vi "CV.vi"(2 "Run uninterrupted?":bool, 3 "Device Category IN:":string(combo)="Short Strip" caption="Device Category:", 4 "Batch No.:":string, 5 "Wafer Serial No.:":string, 6 "Sensor Serial No.:":string) -> (0 "Done!":bool)   [LabVIEW 2018]
doc: "Performs CV measurements according to ATLAS ITk Quality Control Specifications."
uses:
  general_VIs/globals/QC_MeasurementSetup.vi
  general_VIs/globals/QC_RunInformation.vi
  InstrControl/InstrumentSetup.vi
  InstrControl/Switching/Switching.lvclass
  InstrControl/SupplyControl/SupplyControl.lvclass
  InstrControl/LCRControl/LCRControl.lvclass
  InstrControl/ArduinoControl/ArduinoControl.lvclass
  <vilib>/Analysis/NI_AALBase.lvlib
  InstrControl/InstrControl.lvclass
panel:
  out "Frequency [Hz]":i32=1000 format="%#.3p"
  out "Resistance":dbl[](array[numeric]) caption="Res [kOhm]"
  out "Initial volts [V]":dbl format="%.1f"
  out "Final volts [V]":dbl=-700.0 format="%.1f"
  out "step [V]":dbl=10.0 format="%.1f"
  out "step interval [s]":u32=5
  out "Volts":dbl[](array[numeric]) caption="Volts [V]"
  out "Capacitance":dbl[](array[numeric]) caption="Cap [pF]"
  out "Temp.":dbl[](array[numeric]) caption="Temp. [°C]" format="%#.2f"
  out "RH":dbl[](array[numeric]) caption="RH [%]" format="%#.2f"
  out "Cgraph":cluster{"Initial volts":dbl, dbl, dbl[]}(graph)
  in  "Scales":T1(ring)
  in  "Cscale":enum16{"1/C^2 [1/nF^2]", "nF", "pF"}(ring)
  out "positive ramp?":bool
  out "Tab Control":enum32{"CV Setup", "CV Scan"}(tab)
  in  "Switching":string(combo)="LXIPXI Switching"
  in  "Frequency [Hz] Setup":i32=1000 caption="Frequency [Hz]" format="%#.3p"
  in  "LCR Meter":string(combo)="WayneKerr 6440B"
  in  "User:":string(combo)="Graham"
  in  "CV Supply":string(combo)="Keithley 2410"
  in  "Configurations":bool
  in  "Set\ncurrent\nlimit?":bool
  in  "Current \nLimit \n[µA]":dbl=1000.0 min=0.0001 format="%.3f"
  in  "Manufacturer:":string(combo)="Hamamatsu"
  in  "Quit":bool
  in  "Continue":bool
  in  "Temperature":enum16{"Read Arduino", "Enter manually"}(ring)=enum."Enter manually"
  in  "abort":bool
  out "Device Category:":string
  out "Batch:":string
  out "Current Volts:":dbl format="%.2f"
  in  "quit (no save)":bool
  in  "Quit & Save":bool
  out "Bias On/Off:":bool
  out "STATUS 1":string
  out "Initiated:":string
  out "Sensor No.:":string
  out "No of steps":u32
  out "Current reading No.":u32
  out "Last reading at:":string
  # "University of\nCambridge"
  # "Strip Sensor QC: CV"
  # "CV Scan parameters:"
  # "Last 5 readings:"
  # "n-4"
  # "n-3"
  # "n-2"
  # "n-1"
  # "n"
  # "Vertical Scale:"
  # "DUT & Test Description"
  # "Hardware"
  # "DUT & Test Description:"
  # "Current status:"
  # "Rdg No:"
  # "out of"
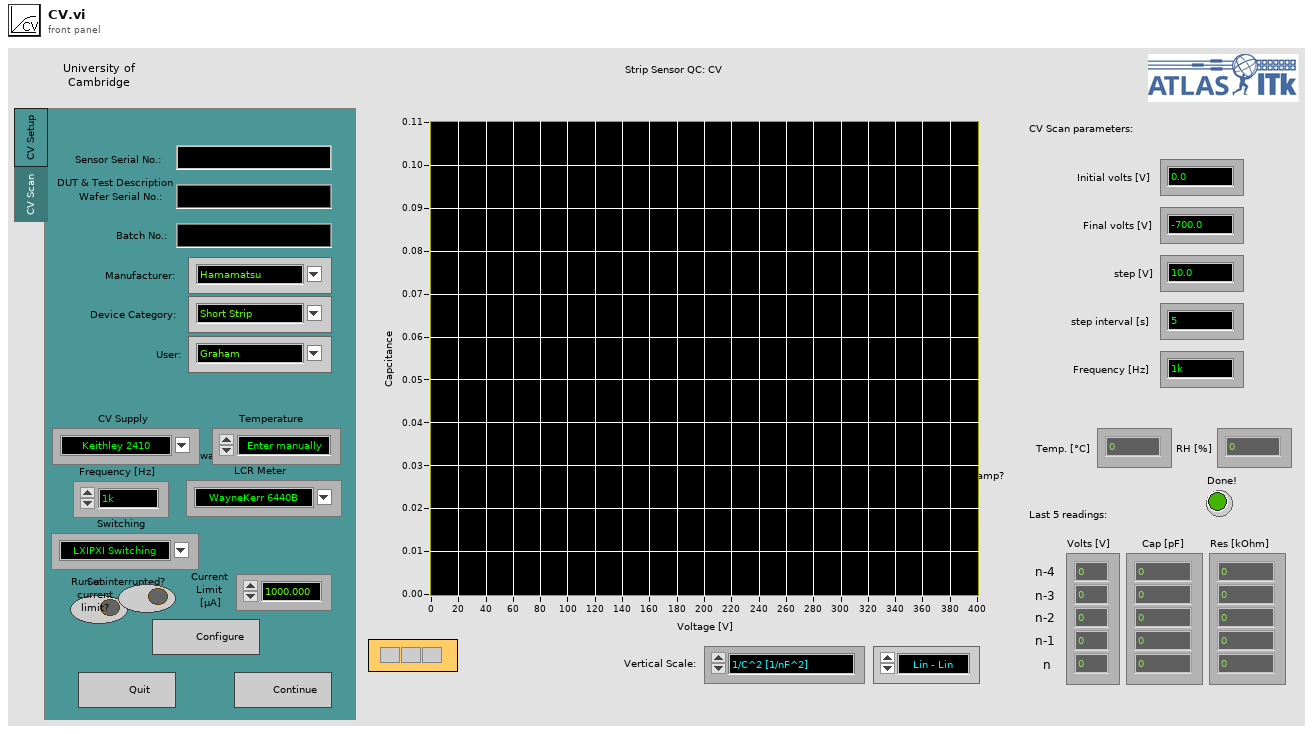
[diagram p1: front panel]
types:
  T1 = enum16{"Lin - Lin", "Log - Lin", "Lin - Log", "Log - log"}
  T2 = enum32{"IV", "CV", "Stability", "Striptest", "Cis", "Ris", "PTP"}
  T3 = enum16{"Reset", "Read Array", "Read Element", "Write Element", "Write Array", "Add Element", "Add Array"}
  T4 = enum16{"Reset", "Ground", "Striptest SMU", "Striptest LCR", "IV", "CV", "Interstrip Cap", "Interstrip Res"}
  T5 = cluster{"Sensor Serial No.:":string, "Wafer Serial No.:":string, "Batch:":string, "Manufacturer:":string, "Device Category:":string, "Database Serial No.:":string, "Initiated:":string, "Test":string, "Instruments used:":string, "Probeplan used:":string, "End of Run comment:":string, "User:":string}
  T6 = cluster{"Institute":string, "Manufacturers":string[], "Devices":string[], "Serialnumbers Lookup DB":string, "Data directory":string, "Backup & screenshot directory":string, "List of known users":string[]}
  T7 = cluster{"Supply":refnum<class "SupplyControl.lvclass">, "LCR":refnum<class "LCRControl.lvclass">, "Initial Voltage [V]":dbl, "Final Voltage [V]":dbl, "Step Size [V]":dbl, "Step Interval [s]":i32, "Number Of Steps":u32, "AC frequency [Hz]":i32, "RC Configuration":u16, "AC amplitude [V]":dbl, "Ramp down steps [V]":dbl, "Ramp down Interval [s]":i32, "Set Current Limit?":bool, "Current Limit [µA]":dbl, "Temperature Readout":enum16{"Read Arduino", "Enter manually"}, "Arduino":refnum<class "ArduinoControl.lvclass">, "Supply Name":string, "LCR Name":string, "V_depletion Limit [V]":dbl, "Switching":refnum<class "Switching.lvclass">}
  T8 = cluster{"VISA address":refnum<visa-resource-name>, "T sensor":enum16{"SHT", "DS"}, "Arduino":refnum<class "ArduinoControl.lvclass">}
  T9 = cluster{"Matrix address":string, "Mux1 address":string, "Mux2 address":string, "Matrix used?":bool, "Switching":refnum<class "Switching.lvclass">, "Matrix X Channels":cluster{"Bias Supply / SMU LO":i32, "Bias Supply / SMU HI":i32, "CV Box LO":i32, "CV Box HI":i32, "CV Box LO IN":i32, "CV Box HI IN":i32, "Volt meter LO":i32, "Volt meter HI":i32, "Mux1 C1":i32, "Mux1 C2":i32, "Mux2 C1":i32, "Mux2 C2":i32}}
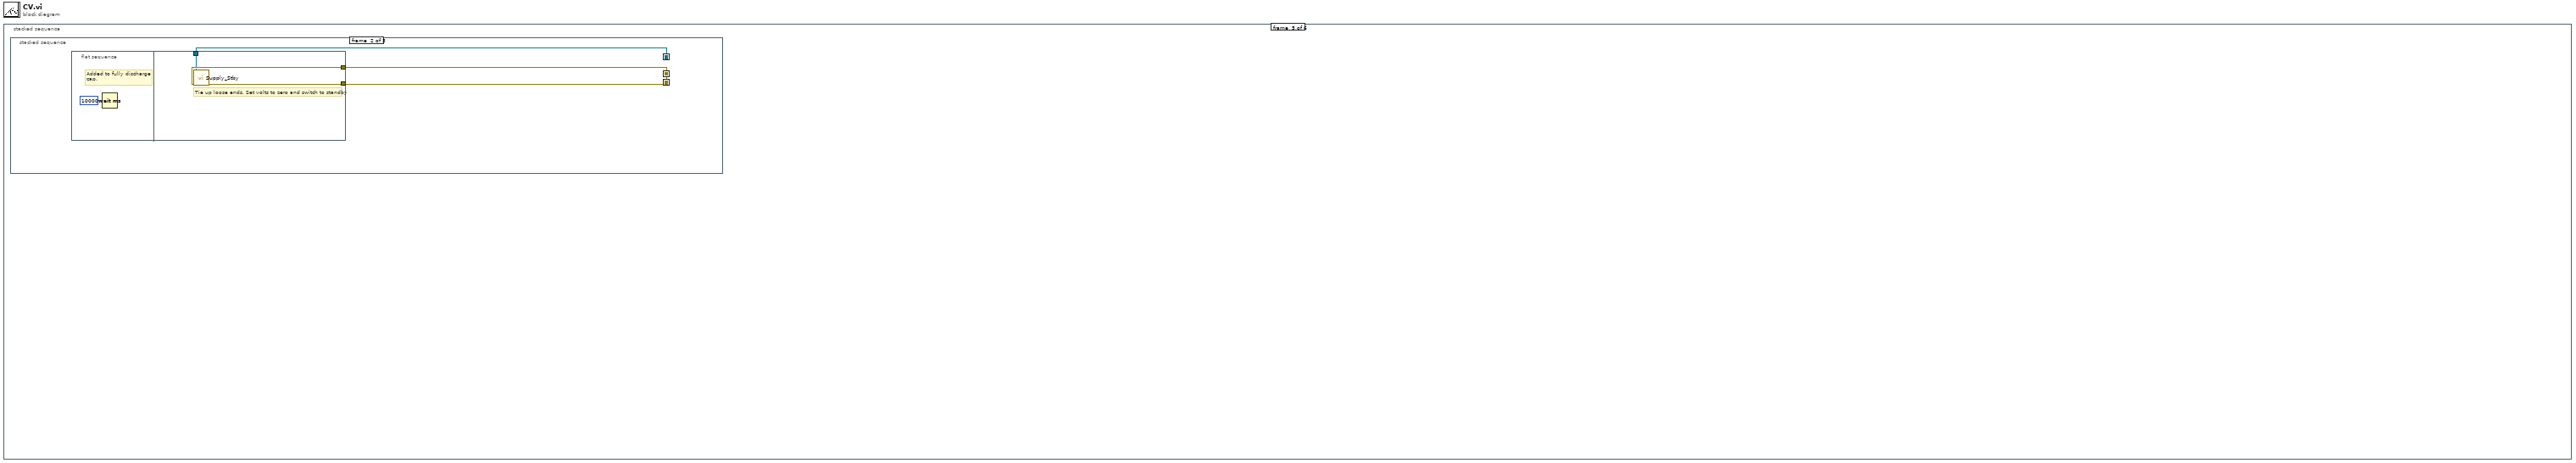
[diagram p0: block diagram]
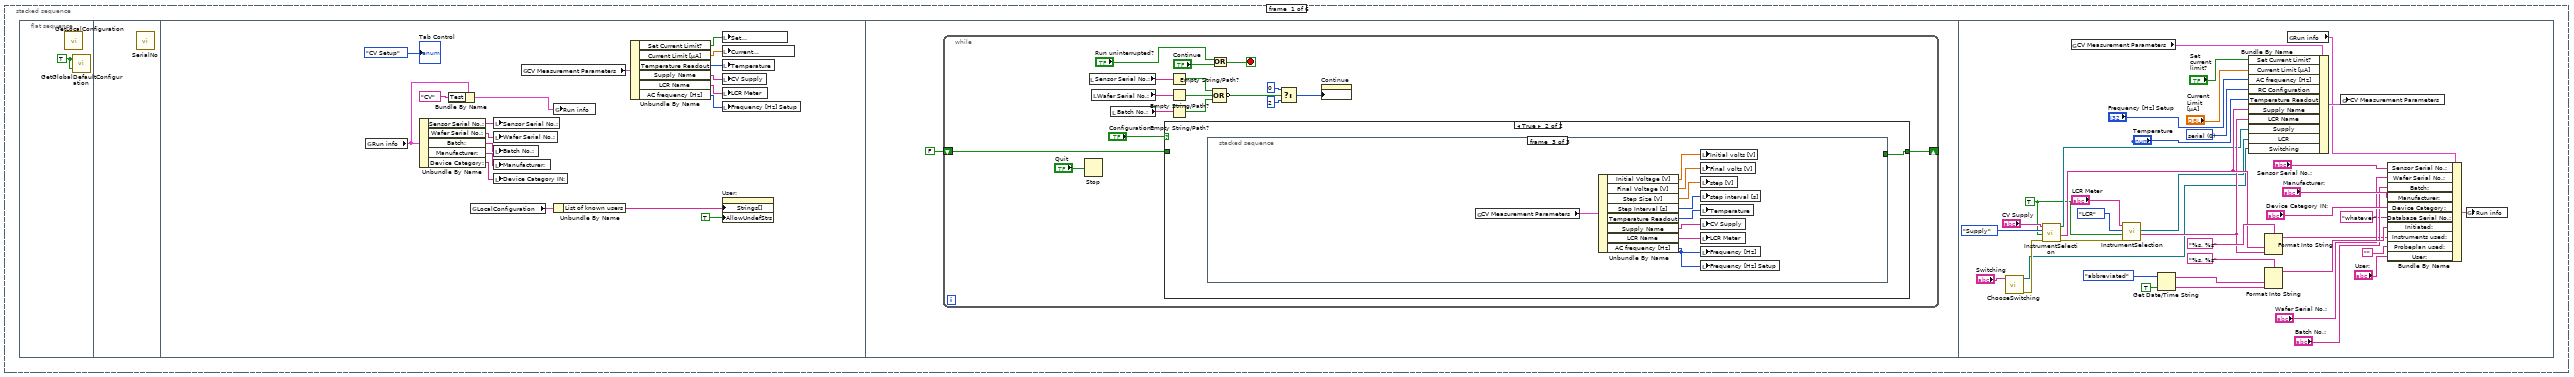
[diagram p2: hidden frame]
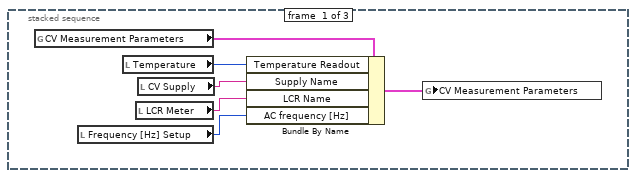
[diagram p4: hidden frame]
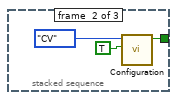
[diagram p5: hidden frame]
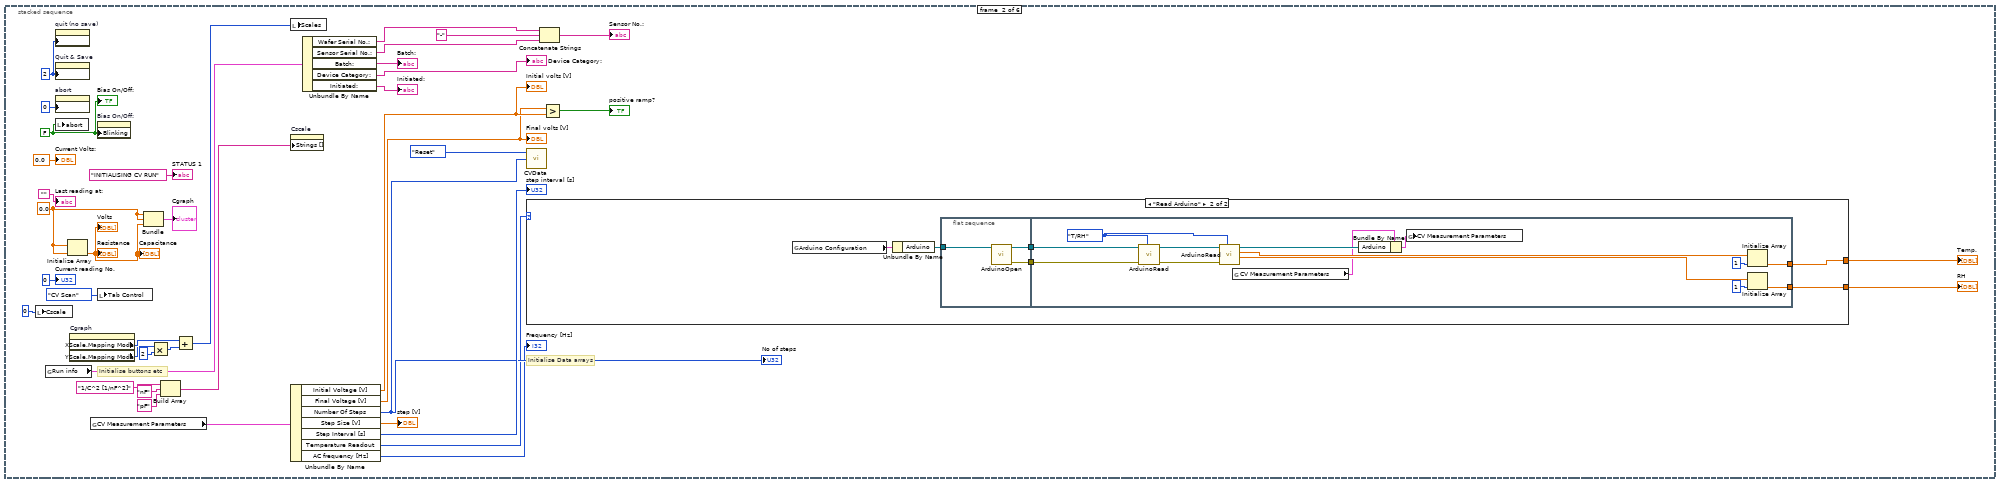
[diagram p6: hidden frame]
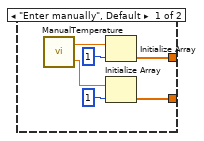
[diagram p7: hidden frame]
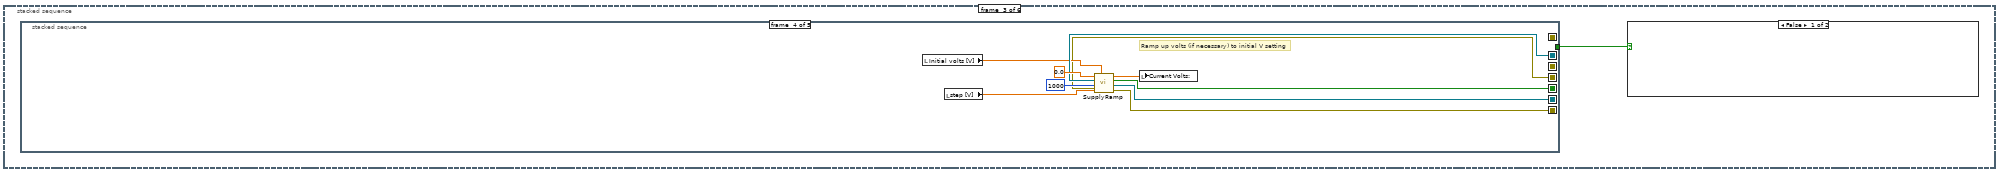
[diagram p8: hidden frame]
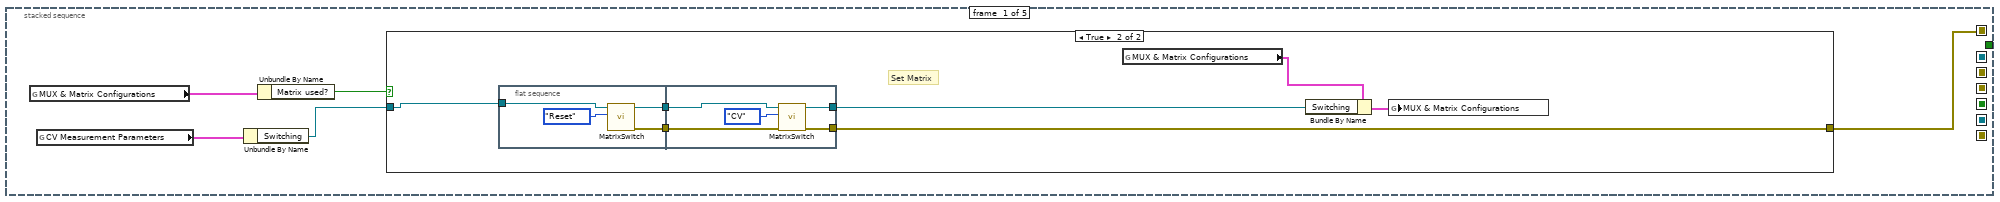
[diagram p9: hidden frame]
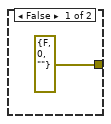
[diagram p10: hidden frame]
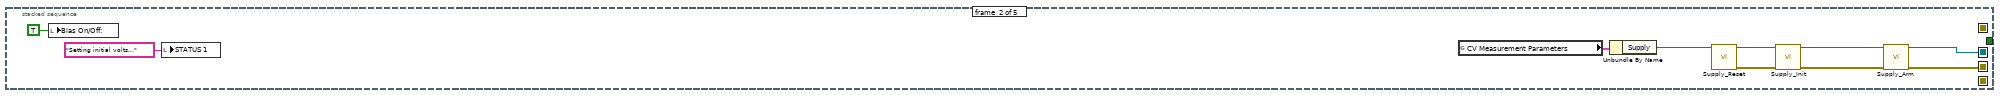
[diagram p11: hidden frame]
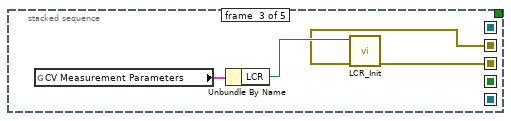
[diagram p12: hidden frame]
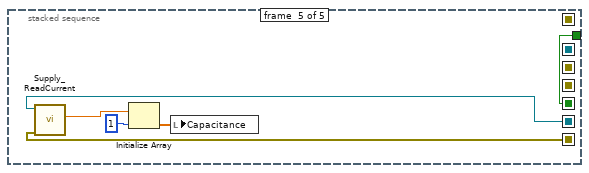
[diagram p13: hidden frame]
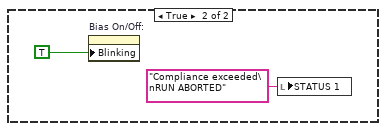
[diagram p14: hidden frame]
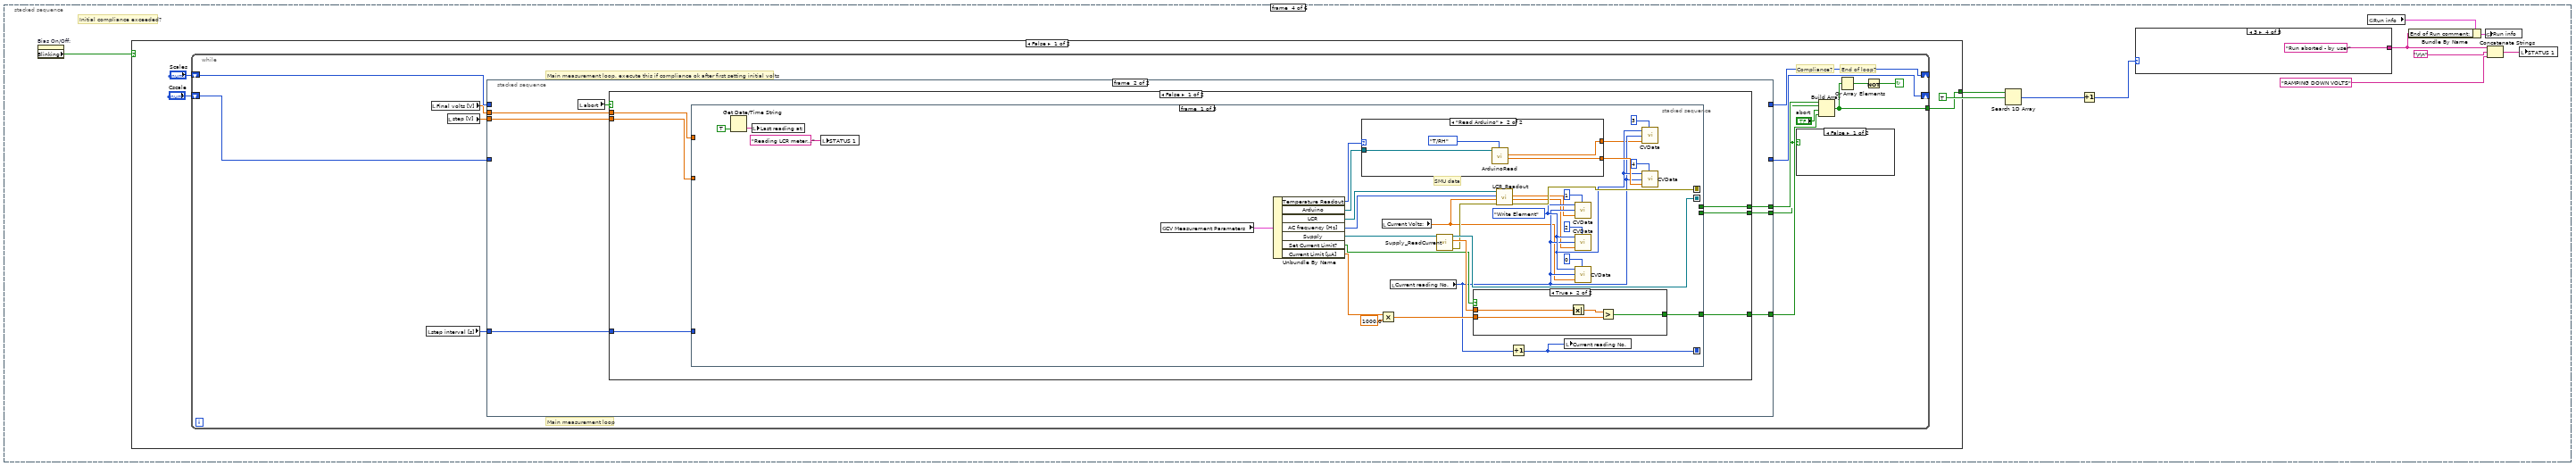
[diagram p15: hidden frame]
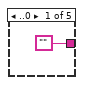
[diagram p16: hidden frame]
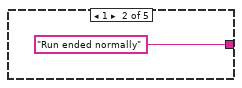
[diagram p17: hidden frame]
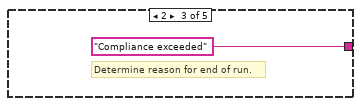
[diagram p18: hidden frame]
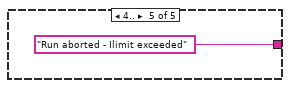
[diagram p19: hidden frame]
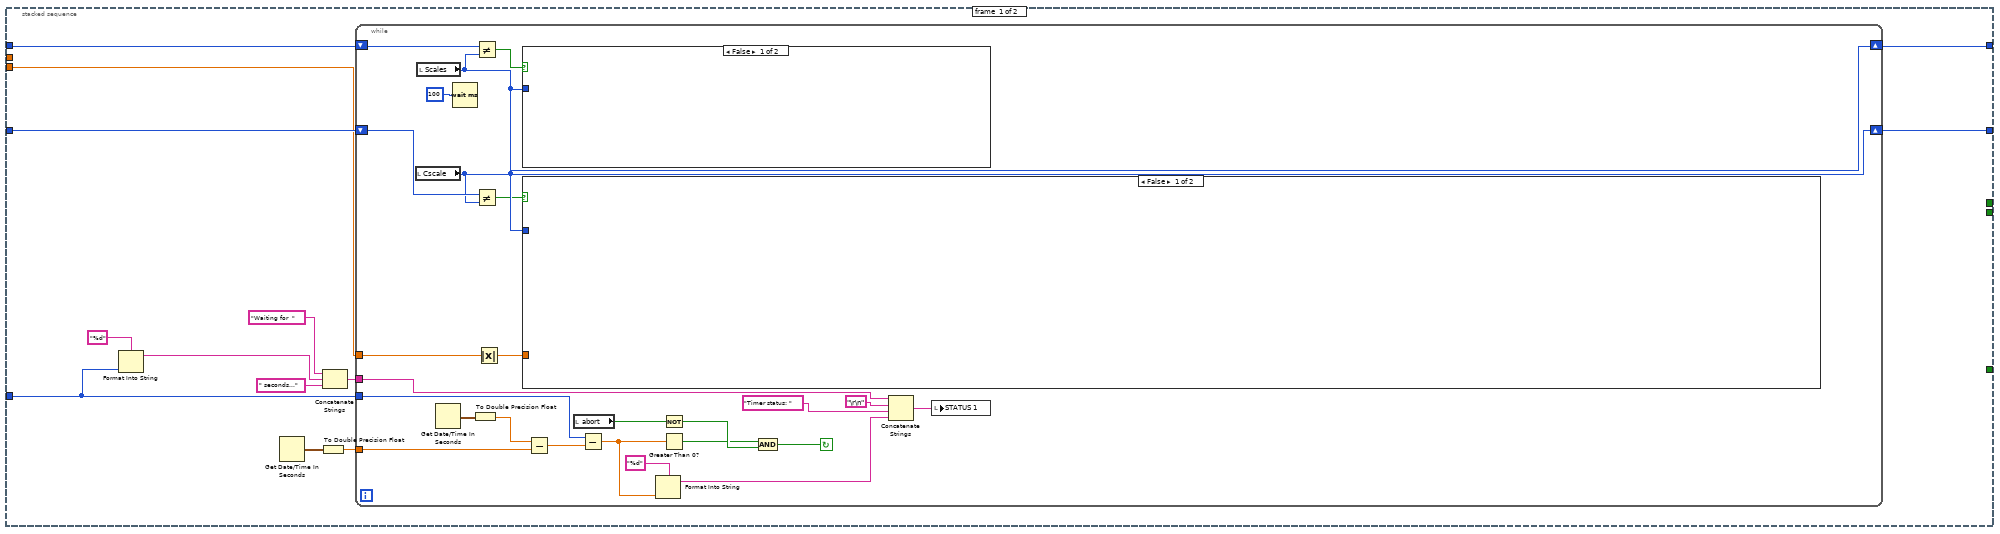
[diagram p20: hidden frame]
diagram:
  n1 = stacked-sequence {
    frame #0 {
      n2 = flat-sequence {
        frame #0 {
          w1 = TRUE
          n3 = call "GetLocalConfiguration.vi"() -> ()  [unwired: 3 in, 1 out]
          n4 = call "GetGlobalDefaultConfiguration.vi"("DO NOT override instruments"=w1, "Read defaults?"=w1) -> ()  [unwired: 1 in, 1 out]
        }
        frame #1 {
          n5 = call "SerialNo.vi"() -> ()  [unwired: 5 in, 1 out]
        }
        frame #2 {
          n6 = global read "QC_RunInformation.vi" "Run info"() -> (w7:T5)
          n7 = Unbundle By Name(w7) -> ("Sensor Serial No.:"=w2:string, "Wafer Serial No.:"=w3:string, "Batch:"=w4:string, "Manufacturer:"=w5:string, "Device Category:"=w6:string)
          n8 = Bundle By Name(cluster=w7, "Test"="CV") -> (w9:T5)
          n9 = global read "QC_RunInformation.vi" "LocalConfiguration"() -> (w15:T6)
          n10 = local write "Sensor Serial No.:"(w2) -> ()
          n11 = local write "Wafer Serial No.:"(w3) -> ()
          n12 = local write "Batch No.:"(w4) -> ()
          n13 = local write "Manufacturer:"(w5) -> ()
          n14 = local write "Device Category IN:"(w6) -> ()
          n15 = global read "QC_MeasurementSetup.vi" "CV Measurement Parameters"() -> (w18:T7)
          n16 = global write "QC_RunInformation.vi" "Run info"(w9) -> ()
          n17 = Unbundle By Name(w15) -> ("List of known users"=w14:string[])
          n18 = Unbundle By Name(w18) -> ("Set Current Limit?"=w17:bool, "Current Limit [µA]"=w16:dbl, "Temperature Readout"=w20:enum16{"Read Arduino", "Enter manually"}, "Supply Name"=w19:string, "LCR Name"=w11:string, "AC frequency [Hz]"=w10:i32)
          n19 = local write "Set\ncurrent\nlimit?"(w17) -> ()
          n20 = local write "Current \nLimit \n[µA]"(w16) -> ()
          n21 = local write "Temperature"(w20) -> ()
          n22 = local write "CV Supply"(w19) -> ()
          n23 = local write "LCR Meter"(w11) -> ()
          n24 = local write "Frequency [Hz] Setup"(w10) -> ()
          n25 = property on="User:" class="CmbBox"("Strings[]"=w14, "AllowUndefStrs"=TRUE) -> ()  [unwired: 2 in, 2 out]
          "Tab Control" <- enum32{"CV Setup", "CV Scan"}."CV Setup" ("Tab Control")
        }
        frame #3 {
          n26 = while {
            shift-right: [w26] -> _
            shift-left: FALSE -> [w25]
            stop <- w22 stop-if-true
            n27 = Stop(stop? (T)="Quit") -> ()
            n28 = local read "Sensor Serial No.:"() -> (w37:string)
            n29 = local read "Wafer Serial No.:"() -> (w36:string)
            n30 = local read "Batch No.:"() -> (w28:string)
            n31 = case shown="True" "Configurations" {
              tunnel: [w39 w40] -> w26
              tunnel: w25 -> [w39 _]
              frame False {
              }
              frame True {
                n32 = stacked-sequence {
                  tunnel: [_ w47 _] -> w40
                  frame #0 {
                    n33 = global read "QC_MeasurementSetup.vi" "CV Measurement Parameters"() -> (w45:T7)
                    n34 = local read "Frequency [Hz] Setup"() -> (w41:i32)
                    n35 = local read "Temperature"() -> (w44:enum16{"Read Arduino", "Enter manually"})
                    n36 = local read "LCR Meter"() -> (w42:string)
                    n37 = local read "CV Supply"() -> (w43:string)
                    n38 = Bundle By Name(cluster=w45, "Temperature Readout"=w44, "Supply Name"=w43, "LCR Name"=w42, "AC frequency [Hz]"=w41) -> (w46:T7)
                    n39 = global write "QC_MeasurementSetup.vi" "CV Measurement Parameters"(w46) -> ()
                  }
                  frame #1 {
                    n40 = call "Configuration.vi"("Open from\nscan VI"=TRUE, "Measurements"=T2."CV") -> ("configured?"=w47:bool)  [unwired: 9 in]
                  }
                  frame #2 {
                    n41 = global read "QC_MeasurementSetup.vi" "CV Measurement Parameters"() -> (w57:T7)
                    n42 = Unbundle By Name(w57) -> ("Initial Voltage [V]"=w51:dbl, "Final Voltage [V]"=w50:dbl, "Step Size [V]"=w52:dbl, "Step Interval [s]"=w53:i32, "Temperature Readout"=w58:enum16{"Read Arduino", "Enter manually"}, "Supply Name"=w55:string, "LCR Name"=w56:string, "AC frequency [Hz]"=w54:i32)
                    n43 = local write "Initial volts [V]"(w51) -> ()
                    n44 = local write "Final volts [V]"(w50) -> ()
                    n45 = local write "step [V]"(w52) -> ()
                    n46 = local write "step interval [s]"(w53) -> ()
                    n47 = local write "Temperature"(w58) -> ()
                    n48 = local write "CV Supply"(w55) -> ()
                    n49 = local write "LCR Meter"(w56) -> ()
                    n50 = local write "Frequency [Hz]"(w54) -> ()
                    n51 = local write "Frequency [Hz] Setup"(w54) -> ()
                  }
                }
              }
            }
            n52 = Empty String/Path?(string/path=w37) -> (empty?=w34:bool)
            n53 = Empty String/Path?(string/path=w36) -> (empty?=w35:bool)
            n54 = Empty String/Path?(string/path=w28) -> (empty?=w27:bool)
            n55 = Or(x="Run uninterrupted?", y="Continue") -> (x .or. y?=w22:bool)
            n56 = Compound Arithmetic op=OR(w34, w35, w27) -> (invert w33:bool)
            n57 = Select(t=0, s=w33, f=2) -> (s? t:f=w30:i32)
            n58 = property on="Continue" class="Bool"("DisabledEnum"=w30) -> ()  [unwired: 2 in, 2 out]
          }
        }
        frame #4 {
          w62 = TRUE
          w75 = u16 0 items=["serial", "parallel"] ("RC Configuration")
          n59 = call "ChooseSwitching.vi"("Instrument name IN"="Switching") -> ("error in (no error) 2"=w60:errorcluster, "Switching.lvclass"=w59:refnum<class "Switching.lvclass">)  [unwired: 9 in]
          n60 = call "InstrumentSelection.vi"("error in (no error)"=w60, "Verify GPIB address"=w62, "Instrument type"=enum16{"Supply", "LCR", "Multimeter"}."Supply", "Instrument name IN"="CV Supply") -> ("error out"=w65:errorcluster, "Instrument name OUT"=w68:string, "Supply"=w64:refnum<class "SupplyControl.lvclass">)  [unwired: 3 in, 2 out]
          n61 = global read "QC_MeasurementSetup.vi" "CV Measurement Parameters"() -> (w95:T7)
          n62 = call "InstrumentSelection.vi"("error in (no error)"=w65, "Verify GPIB address"=w62, "Instrument type"=enum16{"Supply", "LCR", "Multimeter"}."LCR", "Instrument name IN"="LCR Meter") -> ("Instrument name OUT"=w67:string, "LCR"=w63:refnum<class "LCRControl.lvclass">)  [unwired: 3 in, 3 out]
          n63 = Get Date/Time String(date format (0)=enum16{"short", "long", "abbreviated"}."abbreviated", want seconds? (F)=TRUE) -> (date string=w90:string, time string=w89:string)  [unwired: 1 in]
          n64 = Bundle By Name(cluster=w95, "Set Current Limit?"="Set\ncurrent\nlimit?", "Current Limit [µA]"="Current \nLimit \n[µA]", "AC frequency [Hz]"="Frequency [Hz] Setup", "RC Configuration"=w75, "Temperature Readout"="Temperature", "Supply Name"=w68, "LCR Name"=w67, "Supply"=w64, "LCR"=w63, "Switching"=w59) -> (w96:T7)
          n65 = Format Into String(format string="%s, %s", w68, w67) -> (resulting string=w72:string)  [unwired: 2 in, 1 out]
          n66 = Format Into String(format string="%s, %s", w90, w89) -> (resulting string=w85:string)  [unwired: 2 in, 1 out]
          n67 = global read "QC_RunInformation.vi" "Run info"() -> (w87:T5)
          n68 = global write "QC_MeasurementSetup.vi" "CV Measurement Parameters"(w96) -> ()
          n69 = Bundle By Name(cluster=w87, "Sensor Serial No.:"="Sensor Serial No.:", "Wafer Serial No.:"="Wafer Serial No.:", "Batch:"="Batch No.:", "Manufacturer:"="Manufacturer:", "Device Category:"="Device Category IN:", "Database Serial No.:"="whatever", "Initiated:"=w85, "Instruments used:"=w72, "Probeplan used:"="", "User:"="User:") -> (w86:T5)
          n70 = global write "QC_RunInformation.vi" "Run info"(w86) -> ()
        }
      }
    }
    frame #1 {
      w119 = 2
      w126 = 0.0
      w118 = FALSE ("Visible")
      # "Initialise buttons etc"
      # "Initialise Data arrays"
      n71 = local write "Cscale"(u16 0 ("Scale")) -> ()
      n72 = global read "QC_RunInformation.vi" "Run info"() -> (w136:T5)
      n73 = property on="quit (no save)" class="Bool"("DisabledEnum"=w119) -> ()  [unwired: 2 in, 2 out]
      n74 = property on="Quit & Save" class="Bool"("DisabledEnum"=w119) -> ()  [unwired: 2 in, 2 out]
      n75 = property on="abort" class="Bool (strict)"("DisabledEnum"=0) -> ()  [unwired: 2 in, 2 out]
      n76 = local write "abort"(w118) -> ()
      n77 = Initialize Array(w126, w126) -> (w98:dbl[])
      "Volts" <- w98
      "Capacitance" <- w98
      "Resistance" <- w98
      n78 = property on="Cgraph" class="WFGraph (strict)"() -> ("XScale.Mapping Mode"=w111:u8, "YScale.Mapping Mode"=w110:u8)  [unwired: 2 in, 2 out]
      n79 = global read "QC_MeasurementSetup.vi" "CV Measurement Parameters"() -> (w107:T7)
      n80 = property on="Bias On/Off:" class="Bool (strict)"("Blinking"=w118) -> ()  [unwired: 2 in, 2 out]
      n81 = local write "Tab Control"(enum32{"CV Setup", "CV Scan"}."CV Scan" ("Tab Control")) -> ()
      n82 = Bundle(w126, w126, w98) -> (→"Cgraph":cluster{dbl, dbl, dbl[]})  [unwired: 1 in]
      n83 = Multiply(x=w110, y=2) -> (x*y=w113:i32)
      n84 = Build Array("1/C^2 [1/nF^2]", "nF", "pF") -> (w133:string[])
      n85 = Add(x=w111, y=w113) -> (x+y=w109:i32)
      n86 = local write "Scales"(w109) -> ()
      n87 = property on="Cscale" class="Enum (strict)"("Strings []"=w133) -> ()  [unwired: 2 in, 2 out]
      n88 = Unbundle By Name(w107) -> ("Initial Voltage [V]"=w117:dbl, "Final Voltage [V]"=w116:dbl, "Number Of Steps"=w127:u32, "Step Size [V]"=→"step [V]":dbl, "Step Interval [s]"=→"step interval [s]":i32, "Temperature Readout"=w120:enum16{"Read Arduino", "Enter manually"}, "AC frequency [Hz]"=→"Frequency [Hz]":i32)
      "No of steps" <- w127
      "Initial volts [V]" <- w117
      "Final volts [V]" <- w116
      n89 = Unbundle By Name(w136) -> ("Wafer Serial No.:"=w104:string, "Sensor Serial No.:"=w103:string, "Batch:"=→"Batch:":string, "Device Category:"=→"Device Category:":string, "Initiated:"=→"Initiated:":string)
      n90 = call "CVData.vi"("Action"=T3."Reset", "Array Size / Index"=w127) -> ()  [unwired: 3 in, 2 out]
      n91 = case shown="\"Read Arduino\"" w120 {
        tunnel: [w142 w149] -> w123
        tunnel: [w139 w148] -> w108
        frame "Enter manually", Default {
          n92 = call "ManualTemperature.vi"() -> ("Humidity [%] out"=w138:dbl, "Temperature [°C] out"=w143:dbl)
          n93 = Initialize Array(w143, 1) -> (w142:dbl[])
          n94 = Initialize Array(w138, 1) -> (w139:dbl[])
        }
        frame "Read Arduino" {
          n95 = global read "InstrumentSetup.vi" "Arduino Configuration"() -> (w145:T8)
          n96 = Unbundle By Name(w145) -> ("Arduino"=w144:refnum<class "ArduinoControl.lvclass">)
          n97 = flat-sequence {
            tunnel: [w150] -> w147
            tunnel: [w152] -> w146
            tunnel: w144 -> [w151]
            tunnel: [w166] -> w149
            tunnel: [w163] -> w148
            tunnel: w147 -> [w155]
            tunnel: w146 -> [w156]
            frame #0 {
              n98 = call "ArduinoOpen.vi"("ArduinoControl in"=w151) -> ("error out"=w152:errorcluster, "ArduinoControl out"=w150:refnum<class "ArduinoControl.lvclass">)  [unwired: 9 in]
            }
            frame #1 {
              w157 = enum16{"T/RH", "Interlock", "Edgesense"}."T/RH" ("Arduino function")
              n99 = call "ArduinoRead.vi"("Arduino function"=w157, "error in (no error)"=w156, "ArduinoControl in"=w155) -> ("error out"=w153:errorcluster, "ArduinoControl out"=w154:refnum<class "ArduinoControl.lvclass">)  [unwired: 3 in, 4 out]
              n100 = call "ArduinoRead.vi"("Arduino function"=w157, "error in (no error)"=w153, "ArduinoControl in"=w154) -> ("rel. Humidity [%]"=w161:dbl, "Temperature [°C]"=w162:dbl, "ArduinoControl out"=w160:refnum<class "ArduinoControl.lvclass">)  [unwired: 3 in, 3 out]
              n101 = global read "QC_MeasurementSetup.vi" "CV Measurement Parameters"() -> (w159:T7)
              n102 = Bundle By Name(cluster=w159, "Arduino"=w160) -> (w158:T7)
              n103 = global write "QC_MeasurementSetup.vi" "CV Measurement Parameters"(w158) -> ()
              n104 = Initialize Array(w162, 1) -> (w166:dbl[])
              n105 = Initialize Array(w161, 1) -> (w163:dbl[])
            }
          }
        }
      }
      "Temp." <- w123
      "RH" <- w108
      n106 = Concatenate Strings(w104, "-", w103) -> (→"Sensor No.:":string)
      n107 = Greater?(x=w116, y=w117) -> (0:→"positive ramp?":bool)
      "STATUS 1" <- "INITIALISING CV RUN"
      "Bias On/Off:" <- w118
      "Last reading at:" <- ""
      "Current reading No." <- u32 0 ("Current reading No.")
      "Current Volts:" <- 0.0 ("Current Volts:")
    }
    frame #2 {
      n108 = stacked-sequence {
        seq-local: [_ w195 _ _ _] -> [_ _ _ w208 _]
        seq-local: [_ w194 _ _ _] -> [_ _ w201 _ _]
        seq-local: [_ _ _ w209 _] -> [_ _ _ _ w217]
        seq-local: [_ _ _ w207 _] -> [_ _ _ _ w218]
        seq-local: [_ _ _ w206 _] -> [_ _ _ _ w219]
        seq-local: [w170 _ _ _ _] -> [_ _ _ _ _]
        seq-local: [_ _ w200 _ _] -> [_ _ _ w204 _]
        tunnel: [_ _ _ _ w217] -> w167
        frame #0 {
          n109 = global read "InstrumentSetup.vi" "MUX & Matrix Configurations"() -> (w171:T9)
          n110 = global read "QC_MeasurementSetup.vi" "CV Measurement Parameters"() -> (w169:T7)
          n111 = Unbundle By Name(w169) -> ("Switching"=w168:refnum<class "Switching.lvclass">)
          n112 = Unbundle By Name(w171) -> ("Matrix used?"=w172:bool)
          n113 = case shown="True" w172 {
            tunnel: w168 -> [_ w174]
            tunnel: [errorcluster {"status"=FALSE, "code"=0, "source"=""} ("error constant") w175] -> w170
            frame False {
            }
            frame True {
              # "Set Matrix"
              n114 = flat-sequence {
                tunnel: [w184] -> w180
                tunnel: [w183] -> w179
                tunnel: w174 -> [w181]
                tunnel: w180 -> [w189]
                tunnel: w179 -> [w188]
                tunnel: [w187] -> w176
                tunnel: [w186] -> w175
                frame #0 {
                  n115 = call-dynamic "MatrixSwitch.vi"("Action"=T4."Reset", "Switching in"=w181) -> ("error out"=w184:errorcluster, "Switching out"=w183:refnum<class "Switching.lvclass">)  [unwired: 8 in]
                }
                frame #1 {
                  n116 = call-dynamic "MatrixSwitch.vi"("error in (no error)"=w189, "Action"=T4."CV", "Switching in"=w188) -> ("error out"=w186:errorcluster, "Switching out"=w187:refnum<class "Switching.lvclass">)  [unwired: 7 in]
                }
              }
              n117 = global read "InstrumentSetup.vi" "MUX & Matrix Configurations"() -> (w177:T9)
              n118 = Bundle By Name(cluster=w177, "Switching"=w176) -> (w178:T9)
              n119 = global write "InstrumentSetup.vi" "MUX & Matrix Configurations"(w178) -> ()
            }
          }
        }
        frame #1 {
          n120 = local write "Bias On/Off:"(TRUE ("Compliance?")) -> ()
          n121 = local write "STATUS 1"("Setting initial volts..." ("STATUS 1")) -> ()
          n122 = global read "QC_MeasurementSetup.vi" "CV Measurement Parameters"() -> (w193:T7)
          n123 = Unbundle By Name(w193) -> ("Supply"=w190:refnum<class "SupplyControl.lvclass">)
          n124 = call-dynamic "Supply_Reset.vi"("SupplyControl in"=w190) -> ("error out"=w197:errorcluster, "SupplyControl out"=w199:refnum<class "SupplyControl.lvclass">)  [unwired: 9 in]
          n125 = call-dynamic "Supply_Init.vi"("error in (no error)"=w197, "SupplyControl in"=w199) -> ("error out"=w196:errorcluster, "SupplyControl out"=w198:refnum<class "SupplyControl.lvclass">)  [unwired: 8 in]
          n126 = call-dynamic "Supply_Arm.vi"("error in (no error)"=w196, "SupplyControl in"=w198) -> ("error out"=w194:errorcluster, "SupplyControl out"=w195:refnum<class "SupplyControl.lvclass">)  [unwired: 8 in]
        }
        frame #2 {
          n127 = global read "QC_MeasurementSetup.vi" "CV Measurement Parameters"() -> (w203:T7)
          n128 = Unbundle By Name(w203) -> ("LCR"=w202:refnum<class "LCRControl.lvclass">)
          n129 = call-dynamic "LCR_Init.vi"("error in (no error)"=w201, "LCRControl in"=w202) -> ("error out"=w200:errorcluster)  [unwired: 8 in, 1 out]
        }
        frame #3 {
          # "Ramp up volts (if necessary) to initial V setting"
          n130 = local read "Initial volts [V]"() -> (w205:dbl)
          n131 = local read "step [V]"() -> (w210:dbl)
          n132 = call "SupplyRamp.vi"("error in"=w204, "Requested Voltage"=w205, "Step Size"=w210, "Step Delay"=1000, "Supply IN"=w208, "Starting Voltage"=0.0) -> ("error out"=w207:errorcluster, "Supply OUT"=w206:refnum<class "SupplyControl.lvclass">, "Compliance exceeded"=w209:bool, "Current Voltage"=w213:dbl)  [unwired: 2 in]
          n133 = local write "Current Volts:"(w213) -> ()
        }
        frame #4 {
          n134 = call-dynamic "Supply_ReadCurrent.vi"("error in (no error)"=w218, "SupplyControl in"=w219) -> ("Current in nA"=w215:dbl)  [unwired: 7 in, 2 out]
          n135 = Initialize Array(w215, 1) -> (w214:dbl[])
          n136 = local write "Capacitance"(w214) -> ()
        }
      }
      n137 = case shown="False" w167 {
        frame False {
        }
        frame True {
          n138 = property on="Bias On/Off:" class="Bool (strict)"("Blinking"=TRUE) -> ()  [unwired: 2 in, 2 out]
          n139 = local write "STATUS 1"("Compliance exceeded\nRUN ABORTED") -> ()
        }
      }
    }
    frame #3 {
      # "Initial compliance exceeded?"
      n140 = property on="Bias On/Off:" class="Bool (strict)"() -> ("Blinking"=w232:bool)  [unwired: 2 in, 2 out]
      n141 = case shown="False" w232 {
        tunnel: [w240 w487] -> w231
        frame False {
          n142 = while {
            shift-left: "Cscale" -> [w250]
            shift-right: [w249] -> _
            shift-left: "Scales" -> [w251]
            shift-right: [w252] -> _
            tunnel: [w248] -> w240
            stop <- w253 continue-if-true
            # "Main measurement loop"
            # "End of loop?"
            # "Compliance?"
            # "Main measurement loop. execute this if compliance ok after first setting initial volts"
            n143 = local read "step interval [s]"() -> (w245:u32)
            n144 = local read "Final volts [V]"() -> (w246:dbl)
            n145 = local read "step [V]"() -> (w247:dbl)
            n146 = stacked-sequence {
              tunnel: [w267 _] -> w252
              tunnel: w247 -> [w264 w330]
              tunnel: [_ w329] -> w242
              tunnel: w246 -> [_ w328]
              tunnel: w245 -> [w255 w327]
              tunnel: [_ w326] -> w244
              tunnel: w251 -> [w266 _]
              tunnel: w250 -> [w265 _]
              tunnel: [w263 _] -> w249
              tunnel: [_ w324] -> w243
              frame #0 {
                n147 = Format Into String(format string="%d", w255) -> (resulting string=w260:string)  [unwired: 2 in, 1 out]
                n148 = Get Date/Time In Seconds() -> (seconds since 1Jan1904=w257:timestamp)
                n149 = To Double Precision Float(number=w257) -> (double precision float=w258:dbl)
                n150 = Concatenate Strings("Waiting for  ", w260, " seconds...") -> (w256:string)
                n151 = while {
                  tunnel: w264 -> [w276]
                  shift-left: w265 -> [w280]
                  shift-right: [w273] -> w263
                  shift-left: w266 -> [w281]
                  shift-right: [w282] -> w267
                  tunnel: w256 -> [w274]
                  tunnel: w255 -> [w286]
                  tunnel: w258 -> [w287]
                  stop <- w288 continue-if-true
                  n152 = local read "Cscale"() -> (w273:enum16{"1/C^2 [1/nF^2]", "nF", "pF"})
                  n153 = local read "Scales"() -> (w282:T1)
                  n154 = Get Date/Time In Seconds() -> (seconds since 1Jan1904=w272:timestamp)
                  n155 = Wait (ms)(milliseconds to wait=u32 100) -> ()  [unwired: 1 out]
                  n156 = To Double Precision Float(number=w272) -> (double precision float=w292:dbl)
                  n157 = Not Equal?(x=w281, y=w282) -> (x != y?=w283:bool)
                  n158 = Not Equal?(x=w280, y=w273) -> (x != y?=w271:bool)
                  n159 = Absolute Value(x=w276) -> (abs(x)=w275:dbl)
                  n160 = case shown="False" w283 {
                    tunnel: w282 -> [_ w317]
                    frame False {
                    }
                    frame True {
                      n161 = case shown="\"Log - log\".." w317 {
                        tunnel: [w318 1 0 w323] -> w316
                        tunnel: [w318 0 1 w323] -> w315
                        frame .."Lin - Lin" {
                          w318 = 0
                        }
                        frame "Log - Lin" {
                        }
                        frame "Lin - Log" {
                        }
                        frame "Log - log".. {
                          w323 = 1
                        }
                      }
                      n162 = property on="Cgraph" class="WFGraph (strict)"("Y Scale.Mapping Mode"=w315, "YScale.Minimum"=w315) -> ()  [unwired: 2 in, 2 out]
                      n163 = property on="Cgraph" class="WFGraph (strict)"("X Scale.Mapping Mode"=w316) -> ()  [unwired: 2 in, 2 out]
                    }
                  }
                  n164 = case shown="False" w271 {
                    tunnel: w275 -> [_ w304]
                    tunnel: w273 -> [_ w297]
                    frame False {
                    }
                    frame True {
                      n165 = property on="Cgraph" class="WFGraph (strict)"() -> ("YScale.Mapping Mode"=w299:u8)  [unwired: 2 in, 2 out]
                      n166 = local read "Current reading No."() -> (w302:u32)
                      n167 = property on="Cgraph" class="WFGraph (strict)"("YScale.Minimum"=w299) -> ()  [unwired: 2 in, 2 out]
                      n168 = call "CVData.vi"("Action"=T3."Read Array", "Array No."=u32 1 ("Action")) -> ("Array OUT"=w293:dbl[])  [unwired: 3 in, 1 out]
                      n169 = Array Subset(array=w293, index=0, length=w302) -> (w300:dbl[])
                      n170 = Absolute Value(x=w300) -> (abs(x)=w298:dbl[])
                      n171 = case shown="..\"1/C^2 [1/nF^2]\"" w297 {
                        tunnel: [w308 w311 w314] -> w296
                        tunnel: w298 -> [w306 w313 w314]
                        frame .."1/C^2 [1/nF^2]" {
                          n172 = Array Size(array=w306) -> (size(s)=w307:i32)
                          n173 = for {
                            N: w307 -> [_]
                            tunnel: w306 -> [w310] mode=indexing
                            tunnel: [w309] -> w308 mode=indexing
                            n174 = formula code="y=1000000./(x*x);"("x"=w310) -> ("y"=w309:dbl)
                          }
                        }
                        frame "nF" {
                          n175 = Divide(x=w313, y=1000.0) -> (x/y=w311:dbl[])
                        }
                        frame "pF".. {
                        }
                      }
                      n176 = local read "Initial volts [V]"() -> (w303:dbl)
                      n177 = Bundle("Initial volts [V]"=w303, w304, w296) -> (w301:cluster{"Initial volts [V]":dbl, dbl, dbl[]})  [unwired: 1 in]
                      n178 = local write "Cgraph"(w301) -> ()
                    }
                  }
                  n179 = Subtract(x=w292, y=w287) -> (x-y=w269:dbl)
                  n180 = local read "abort"() -> (w285:bool)
                  n181 = Subtract(x=w286, y=w269) -> (x-y=w268:dbl)
                  n182 = Format Into String(format string="%d", w268) -> (resulting string=w290:string)  [unwired: 2 in, 1 out]
                  n183 = Not(x=w285) -> (.not. x?=w291:bool)
                  n184 = Greater Than 0?(x=w268) -> (x > 0?=w270:bool)
                  n185 = And(x=w270, y=w291) -> (x .and. y?=w288:bool)
                  n186 = Concatenate Strings(w274, "\r\n", "Timer status: ", w290) -> (w284:string)
                  n187 = local write "STATUS 1"(w284) -> ()
                }
              }
              frame #1 {
                n188 = local read "abort"() -> (w325:bool)
                n189 = case shown="False" w325 {
                  tunnel: [w336 w484] -> w326
                  tunnel: w327 -> [w335 _]
                  tunnel: w328 -> [w334 _]
                  tunnel: [w332 w484] -> w329
                  tunnel: w330 -> [w333 _]
                  tunnel: [w331 w484] -> w324
                  frame False {
                    n190 = stacked-sequence {
                      seq-local: [w362 _ _] -> [_ w386 _]
                      seq-local: [w361 _ _] -> [_ _ w453]
                      seq-local: [w348 _ _] -> [_ _ w454]
                      tunnel: w333 -> [_ w398 w459]
                      tunnel: w334 -> [_ _ w450]
                      tunnel: [_ _ w457] -> w336
                      tunnel: [_ _ w456] -> w332
                      tunnel: w335 -> [_ _ _]
                      tunnel: [w364 _ _] -> w331
                      frame #0 {
                        w345 = T3."Write Element" ("Action")
                        # "SMU data"
                        n191 = Get Date/Time String(want seconds? (F)=TRUE) -> (time string=w363:string)  [unwired: 2 in, 1 out]
                        n192 = local write "Last reading at:"(w363) -> ()
                        n193 = local write "STATUS 1"("Reading LCR meter..." ("status")) -> ()
                        n194 = global read "QC_MeasurementSetup.vi" "CV Measurement Parameters"() -> (w360:T7)
                        n195 = Unbundle By Name(w360) -> ("Temperature Readout"=w339:enum16{"Read Arduino", "Enter manually"}, "Arduino"=w338:refnum<class "ArduinoControl.lvclass">, "LCR"=w354:refnum<class "LCRControl.lvclass">, "AC frequency [Hz]"=w340:i32, "Supply"=w355:refnum<class "SupplyControl.lvclass">, "Set Current Limit?"=w359:bool, "Current Limit [µA]"=w357:dbl)
                        n196 = case shown="\"Read Arduino\"" w339 {
                          tunnel: [w371 w374] -> w342
                          tunnel: [w368 w377] -> w347
                          tunnel: w338 -> [_ w376]
                          frame "Enter manually", Default {
                            n197 = local read "Temp."() -> (w373:dbl[])
                            n198 = local read "RH"() -> (w369:dbl[])
                            n199 = Index Array(array=w369, index=0) -> (element=w368:dbl)
                            n200 = Index Array(array=w373, index=0) -> (element=w371:dbl)
                          }
                          frame "Read Arduino" {
                            n201 = call "ArduinoRead.vi"("Arduino function"=enum16{"T/RH", "Interlock", "Edgesense"}."T/RH", "ArduinoControl in"=w376) -> ("rel. Humidity [%]"=w377:dbl, "Temperature [°C]"=w374:dbl)  [unwired: 4 in, 4 out]
                          }
                        }
                        n202 = Multiply(x=w357, y=1000.0) -> (x*y=w356:dbl)
                        n203 = local read "Current Volts:"() -> (w337:dbl)
                        n204 = local read "Current reading No."() -> (w344:u32)
                        n205 = call-dynamic "Supply_ReadCurrent.vi"("SupplyControl in"=w355) -> ("error out"=w349:errorcluster, "Current in nA"=w365:dbl, "SupplyControl out"=w361:refnum<class "SupplyControl.lvclass">)  [unwired: 8 in]
                        n206 = case shown="True" w359 {
                          tunnel: w365 -> [_ w382]
                          tunnel: w356 -> [_ w380]
                          tunnel: [FALSE w379] -> w364
                          frame False {
                          }
                          frame True {
                            n207 = Absolute Value(x=w382) -> (abs(x)=w381:dbl)
                            n208 = Greater?(x=w381, y=w380) -> (0:w379:bool)
                          }
                        }
                        n209 = call-dynamic "LCR_Readout.vi"("error in (no error)"=w349, "Current Voltage"=w337, "Frequency in Hz"=w340, "LCRControl in"=w354) -> ("error out"=w348:errorcluster, "Resistance in Ohm"=w343:dbl, "Capacitance in pF"=w341:dbl)  [unwired: 4 in, 1 out]
                        n210 = Increment(x=w344) -> (x+1=w362:u32)
                        n211 = local write "Current reading No."(w362) -> ()
                        n212 = call "CVData.vi"("Action"=w345, "Array No."=u32 1, "Array Size / Index"=w344, "Data IN"=w341) -> ()  [unwired: 1 in, 2 out]
                        n213 = call "CVData.vi"("Action"=w345, "Array No."=u32 2, "Array Size / Index"=w344, "Data IN"=w343) -> ()  [unwired: 1 in, 2 out]
                        n214 = call "CVData.vi"("Action"=w345, "Array No."=0, "Array Size / Index"=w344, "Data IN"=w337) -> ()  [unwired: 1 in, 2 out]
                        n215 = call "CVData.vi"("Action"=w345, "Array No."=u32 3, "Array Size / Index"=w344, "Data IN"=w342) -> ()  [unwired: 1 in, 2 out]
                        n216 = call "CVData.vi"("Action"=w345, "Array No."=u32 4, "Array Size / Index"=w344, "Data IN"=w347) -> ()  [unwired: 1 in, 2 out]
                      }
                      frame #1 {
                        w395 = u32 5 ("y")
                        # "Update plots"
                        n217 = property on="Cgraph" class="WFGraph (strict)"() -> ("YScale.Mapping Mode"=w387:u8)  [unwired: 2 in, 2 out]
                        n218 = Greater?(x=w386, y=w395) -> (0:w394:bool)
                        n219 = case shown="True" w394 {
                          tunnel: w386 -> [w403 w406]
                          tunnel: w395 -> [_ w405]
                          tunnel: [w403 w405] -> w393
                          tunnel: [0 w404] -> w391
                          frame False {
                          }
                          frame True {
                            n220 = Subtract(x=w406, y=w405) -> (x-y=w404:u32)
                          }
                        }
                        n221 = property on="Cgraph" class="WFGraph (strict)"("YScale.Minimum"=w387) -> ()  [unwired: 2 in, 2 out]
                        n222 = call "CVData.vi"("Action"=T3."Read Array", "Array No."=1) -> ("Array OUT"=w384:dbl[])  [unwired: 3 in, 1 out]
                        n223 = Array Subset(array=w384, index=0, length=w386) -> (w390:dbl[])
                        n224 = Absolute Value(x=w390) -> (abs(x)=w389:dbl[])
                        n225 = local read "Cscale"() -> (w396:enum16{"1/C^2 [1/nF^2]", "nF", "pF"})
                        n226 = case shown="..\"1/C^2 [1/nF^2]\"" w396 {
                          tunnel: [w439 w442 w445] -> w401
                          tunnel: w389 -> [w437 w444 w445]
                          frame .."1/C^2 [1/nF^2]" {
                            n227 = Array Size(array=w437) -> (size(s)=w438:i32)
                            n228 = for {
                              N: w438 -> [_]
                              tunnel: w437 -> [w441] mode=indexing
                              tunnel: [w440] -> w439 mode=indexing
                              n229 = formula code="y=1000000./(x*x);"("x"=w441) -> ("y"=w440:dbl)
                            }
                          }
                          frame "nF" {
                            n230 = Divide(x=w444, y=1000.0) -> (x/y=w442:dbl[])
                          }
                          frame "pF".. {
                          }
                        }
                        n231 = for {
                          N: 5 -> [_]
                          tunnel: w393 -> [w412]
                          tunnel: w391 -> [w411]
                          tunnel: w386 -> [w410]
                          i -> [w408]
                          n232 = call "CVData.vi"("Action"=T3."Read Array", "Array No."=w408) -> ("Array OUT"=w407:dbl[])  [unwired: 3 in, 1 out]
                          n233 = case shown="2" w408 {
                            tunnel: w412 -> [w415 w419 w424 _ _]
                            tunnel: w411 -> [w416 w420 w425 _ _]
                            tunnel: w407 -> [w414 w418 w426 w430 w435]
                            tunnel: w410 -> [_ _ _ w428 w433]
                            frame ..0 {
                              n234 = Array Subset(array=w414, index=w416, length=w415) -> (w413:dbl[])
                              n235 = local write "Volts"(w413) -> ()
                            }
                            frame 1 {
                              n236 = Array Subset(array=w418, index=w420, length=w419) -> (w417:dbl[])
                              n237 = local write "Capacitance"(w417) -> ()
                            }
                            frame 2 {
                              n238 = Array Subset(array=w426, index=w425, length=w424) -> (w423:dbl[])
                              n239 = Multiply(x=w423, y=0.001) -> (x*y=w422:dbl[])
                              n240 = local write "Resistance"(w422) -> ()
                            }
                            frame 3 {
                              n241 = Decrement(x=w428) -> (x-1=w427:u32)
                              n242 = Array Subset(array=w430, index=w427, length=1) -> (w429:dbl[])
                              n243 = local write "Temp."(w429) -> ()
                            }
                            frame 4.. {
                              n244 = Decrement(x=w433) -> (x-1=w432:u32)
                              n245 = Array Subset(array=w435, index=w432, length=1) -> (w434:dbl[])
                              n246 = local write "RH"(w434) -> ()
                            }
                          }
                        }
                        n247 = Absolute Value(x=w398) -> (abs(x)=w397:dbl)
                        n248 = local read "Initial volts [V]"() -> (w399:dbl)
                        n249 = Bundle("Initial volts [V]"=w399, w397, w401) -> (w388:cluster{"Initial volts [V]":dbl, dbl, dbl[]})  [unwired: 1 in]
                        n250 = local write "Cgraph"(w388) -> ()
                      }
                      frame #2 {
                        # "Increment volts and check for end of loop"
                        n251 = local read "positive ramp?"() -> (w455:bool)
                        n252 = local read "Current Volts:"() -> (w451:dbl)
                        n253 = case shown="True" w455 {
                          tunnel: w450 -> [w462 w466]
                          tunnel: w459 -> [w463 w469]
                          tunnel: [w461 w468] -> w446
                          tunnel: [w460 w465] -> w458
                          tunnel: w451 -> [w464 w467]
                          frame False {
                            n254 = Subtract(x=w464, y=w463) -> (x-y=w460:dbl)
                            n255 = Greater Or Equal?(x=w460, y=w462) -> (x >= y?=w461:bool)
                          }
                          frame True {
                            n256 = Add(x=w467, y=w469) -> (x+y=w465:dbl)
                            n257 = Less Or Equal?(x=w465, y=w466) -> (x <= y?=w468:bool)
                          }
                        }
                        n258 = Quotient & Remainder(x=w451, y=w450) -> (x-y*floor(x/y)=w452:dbl, floor(x/y)=w449:dbl)
                        n259 = Not Equal To 0?(x=w452) -> (x != 0?=w447:bool)
                        n260 = Equal To 0?(x=w449) -> (x = 0?=w448:bool)
                        n261 = Or(x=w447, y=w448) -> ()  [unwired: 1 out]
                        n262 = case shown="True" w446 {
                          tunnel: w458 -> [_ w480]
                          tunnel: [TRUE FALSE] -> w457
                          tunnel: [FALSE w481] -> w456
                          tunnel: w451 -> [_ w478]
                          tunnel: w454 -> [_ w477]
                          tunnel: w453 -> [_ w476]
                          frame False {
                          }
                          frame True {
                            n263 = local read "step [V]"() -> (w474:dbl)
                            n264 = local write "STATUS 1"("Incrementing volts.") -> ()
                            n265 = call "SupplyRamp.vi"("error in"=w477, "Requested Voltage"=w480, "Step Size"=w474, "Step Delay"=100, "Supply IN"=w476, "Starting Voltage"=w478) -> ("error out"=w472:errorcluster, "Compliance exceeded"=w481:bool, "Current Voltage"=w475:dbl)  [unwired: 2 in, 1 out]
                            n266 = property on="Bias On/Off:" class="Bool (strict)"("Blinking"=w481) -> ()  [unwired: 2 in, 2 out]
                            n267 = case shown="No Error" w472 {
                              tunnel: w475 -> [w483 _]
                              frame No Error {
                                n268 = local write "Current Volts:"(w483) -> ()
                              }
                              frame Error {
                              }
                            }
                          }
                        }
                      }
                    }
                  }
                  frame True {
                    w484 = FALSE
                  }
                }
              }
            }
            n269 = case shown="False" w242 {
              frame False {
              }
              frame True {
                n270 = property on="Bias On/Off:" class="Bool (strict)"("Blinking"=TRUE) -> ()  [unwired: 2 in, 2 out]
              }
            }
            n271 = Build Array(w244, w242, "abort", w243) -> (w248:bool[])
            n272 = Or Array Elements(Boolean array=w248) -> (logical OR=w254:bool)
            n273 = Not(x=w254) -> (.not. x?=w253:bool)
          }
        }
        frame True {
          w486 = FALSE
          # "compliance was exceeded when first voltage applied."
          # "Flag compliance as reason for end of run"
          n274 = local write "STATUS 1"("Run aborted - compliance exceeded.") -> ()
          n275 = Build Array(w486, TRUE, w486, w486) -> (w487:bool[])
        }
      }
      n276 = Search 1D Array(1D array=w231, element=TRUE) -> (index of element=w229:i32)  [unwired: 1 in]
      n277 = Increment(x=w229) -> (x+1=w228:i32)
      n278 = case shown="3" w228 {
        tunnel: ["" "Run ended normally" "Compliance exceeded" "Run aborted - by user" "Run aborted - Ilimit exceeded"] -> w223
        frame ..0 {
        }
        frame 1 {
        }
        frame 2 {
          # "Determine reason for end of run."
        }
        frame 3 {
        }
        frame 4.. {
        }
      }
      n279 = global read "QC_RunInformation.vi" "Run info"() -> (w227:T5)
      n280 = Bundle By Name(cluster=w227, "End of Run comment:"=w223) -> (w222:T5)
      n281 = global write "QC_RunInformation.vi" "Run info"(w222) -> ()
      n282 = Concatenate Strings(w223, "\r\n", "RAMPING DOWN VOLTS") -> (w226:string)
      n283 = local write "STATUS 1"(w226) -> ()
    }
    frame #4 {
      n284 = stacked-sequence {
        seq-local: [w492 _ _ _ _] -> [_ w503 _ _ _]
        seq-local: [w491 _ _ _ _] -> [_ w502 _ _ _]
        seq-local: [_ w501 _ _ _] -> [_ _ w510 _ _]
        frame #0 {
          # "Ramp down volts now"
          n285 = global read "QC_MeasurementSetup.vi" "CV Measurement Parameters"() -> (w495:T7)
          n286 = Unbundle By Name(w495) -> ("Supply"=w490:refnum<class "SupplyControl.lvclass">, "Ramp down steps [V]"=w494:dbl, "Ramp down Interval [s]"=w493:i32)
          n287 = Multiply(x=w493, y=1000) -> (x*y=w497:i32)
          n288 = local read "Current Volts:"() -> (w500:dbl)
          n289 = call "SupplyRamp.vi"("Requested Voltage"=0.0, "Step Size"=w494, "Step Delay"=w497, "Supply IN"=w490, "Starting Voltage"=w500) -> ("error out"=w492:errorcluster, "Supply OUT"=w491:refnum<class "SupplyControl.lvclass">, "Current Voltage"=w498:dbl)  [unwired: 3 in, 1 out]
          n290 = local write "Current Volts:"(w498) -> ()
        }
        frame #1 {
          n291 = flat-sequence {
            tunnel: w503 -> [w507]
            tunnel: w502 -> [w506]
            tunnel: [w505] -> w501
            frame #0 {
              # "Added to fully discharge \ncap."
              n292 = Wait (ms)(milliseconds to wait=u32 10000) -> ()  [unwired: 1 out]
            }
            frame #1 {
              # "Tie up loose ends. Set volts to zero and switch to standby"
              n293 = call-dynamic "Supply_Stby.vi"("error in (no error)"=w507, "SupplyControl in"=w506) -> ("error out"=w505:errorcluster)  [unwired: 8 in, 1 out]
            }
          }
        }
        frame #2 {
          n294 = global read "QC_MeasurementSetup.vi" "CV Measurement Parameters"() -> (w509:T7)
          n295 = global read "InstrumentSetup.vi" "MUX & Matrix Configurations"() -> (w511:T9)
          n296 = Unbundle By Name(w509) -> ("Switching"=w508:refnum<class "Switching.lvclass">)
          n297 = Unbundle By Name(w511) -> ("Matrix used?"=w512:bool)
          n298 = case shown="True" w512 {
            tunnel: w508 -> [_ w517]
            tunnel: w510 -> [_ w516]
            frame False {
            }
            frame True {
              n299 = call-dynamic "MatrixSwitch.vi"("error in (no error)"=w516, "Action"=T4."Reset", "Switching in"=w517) -> ("error out"=w513:errorcluster, "Switching out"=w514:refnum<class "Switching.lvclass">)  [unwired: 7 in]
              n300 = call-dynamic "Close.vi"("error in (no error)"=w513, "Switching in"=w514) -> ()  [unwired: 8 in, 2 out]
            }
          }
        }
        frame #3 {
          w522 = 0
          n301 = local write "Bias On/Off:"(FALSE ("Visible")) -> ()
          n302 = local write "Current Volts:"(0.0 ("Current Volts:")) -> ()
          n303 = property on="Quit & Save" class="Bool"("DisabledEnum"=w522) -> ()  [unwired: 2 in, 2 out]
          n304 = property on="quit (no save)" class="Bool"("DisabledEnum"=w522) -> ()  [unwired: 2 in, 2 out]
          n305 = property on="abort" class="Bool (strict)"("DisabledEnum"=2) -> ()  [unwired: 2 in, 2 out]
          n306 = local write "STATUS 1"("Run finished. \nSave data?" ("STATUS 1")) -> ()
        }
        frame #4 {
          n307 = Current VI's Path() -> (path=w524:path)
          n308 = call "SaveJPEG.vi"("Test"="CV", "File Path Control"=w524) -> ()  [unwired: 1 in, 2 out]
        }
      }
    }
    frame #5 {
      # "Loop and await decision on whether to save or junk data"
      n309 = local read "Cscale"() -> (w534:enum16{"1/C^2 [1/nF^2]", "nF", "pF"})
      n310 = local read "Scales"() -> (w535:T1)
      n311 = global read "QC_MeasurementSetup.vi" "CV Measurement Parameters"() -> (w533:T7)
      n312 = while {
        shift-left: w534 -> [w583]
        shift-right: [w582] -> _
        shift-left: w535 -> [w585]
        shift-right: [w584] -> _
        tunnel: ["Quit & Save"] -> w537
        tunnel: ["quit (no save)"] -> w536
        stop <- w580 continue-if-true
        n313 = local read "Cscale"() -> (w582:enum16{"1/C^2 [1/nF^2]", "nF", "pF"})
        n314 = local read "Scales"() -> (w584:T1)
        n315 = Not Equal?(x=w585, y=w584) -> (x != y?=w578:bool)
        n316 = Not Equal?(x=w583, y=w582) -> (x != y?=w577:bool)
        n317 = case shown="True" w578 {
          tunnel: w584 -> [_ w612]
          frame False {
          }
          frame True {
            n318 = case shown="..\"Lin - Lin\"" w612 {
              tunnel: [w613 1 0 w618] -> w611
              tunnel: [w613 0 1 w618] -> w610
              frame .."Lin - Lin" {
                w613 = 0
              }
              frame "Log - Lin" {
              }
              frame "Lin - Log" {
              }
              frame "Log - log".. {
                w618 = 1
              }
            }
            n319 = property on="Cgraph" class="WFGraph (strict)"("X Scale.Mapping Mode"=w611) -> ()  [unwired: 2 in, 2 out]
            n320 = property on="Cgraph" class="WFGraph (strict)"("Y Scale.Mapping Mode"=w610, "YScale.Minimum"=w610) -> ()  [unwired: 2 in, 2 out]
          }
        }
        n321 = case shown="True" w577 {
          tunnel: w582 -> [_ w590]
          frame False {
          }
          frame True {
            n322 = property on="Cgraph" class="WFGraph (strict)"() -> ("YScale.Mapping Mode"=w593:u8)  [unwired: 2 in, 2 out]
            n323 = property on="Cgraph" class="WFGraph (strict)"("YScale.Minimum"=w593) -> ()  [unwired: 2 in, 2 out]
            n324 = global read "QC_MeasurementSetup.vi" "CV Measurement Parameters"() -> (w592:T7)
            n325 = Unbundle By Name(w592) -> ("Initial Voltage [V]"=w595:dbl, "Step Size [V]"=w597:dbl, "Number Of Steps"=w594:u32)
            n326 = call "CVData.vi"("Action"=T3."Read Array", "Array No."=u32 1 ("Action")) -> ("Array OUT"=w586:dbl[])  [unwired: 3 in, 1 out]
            n327 = Array Subset(array=w586, index=0, length=w594) -> (w598:dbl[])
            n328 = Absolute Value(x=w598) -> (abs(x)=w591:dbl[])
            n329 = case shown="..\"1/C^2 [1/nF^2]\"" w590 {
              tunnel: [w603 w606 w609] -> w589
              tunnel: w591 -> [w601 w608 w609]
              frame .."1/C^2 [1/nF^2]" {
                n330 = Array Size(array=w601) -> (size(s)=w602:i32)
                n331 = for {
                  N: w602 -> [_]
                  tunnel: w601 -> [w605] mode=indexing
                  tunnel: [w604] -> w603 mode=indexing
                  n332 = formula code="y=1000000./(x*x);"("x"=w605) -> ("y"=w604:dbl)
                }
              }
              frame "nF" {
                n333 = Divide(x=w608, y=1000.0) -> (x/y=w606:dbl[])
              }
              frame "pF".. {
              }
            }
            n334 = Absolute Value(x=w597) -> (abs(x)=w596:dbl)
            n335 = Bundle("Initial Voltage [V]"=w595, w596, w589) -> (w599:cluster{"Initial Voltage [V]":dbl, dbl, dbl[]})  [unwired: 1 in]
            n336 = local write "Cgraph"(w599) -> ()
          }
        }
        n337 = Not Or(1:"quit (no save)", 2:"Quit & Save") -> (0:w580:bool)
      }
      n338 = Unbundle By Name(w533) -> ("Temperature Readout"=w532:enum16{"Read Arduino", "Enter manually"}, "Arduino"=w526:refnum<class "ArduinoControl.lvclass">)
      n339 = case shown="\"Read Arduino\"" w532 {
        tunnel: w526 -> [_ w576]
        frame "Enter manually", Default {
        }
        frame "Read Arduino" {
          n340 = call "ArduinoClose.vi"("ArduinoControl in"=w576) -> ()  [unwired: 9 in, 2 out]
        }
      }
      n341 = case shown="True" w536 {
        tunnel: [FALSE w620] -> w538
        frame False {
        }
        frame True {
          n342 = Two Button Dialog(message="Are you sure you don't want to save the data?", 1:"Quit" ("F button name (\"Cancel\")"), 2:"Save data" ("T button name (\"OK\")")) -> (T button?=w620:bool)
        }
      }
      n343 = Or(x=w537, y=w538) -> (x .or. y?=w531:bool)
      n344 = flat-sequence {
        tunnel: w531 -> [w539]
        tunnel: [w539] -> w527
        tunnel: [TRUE] -> w525
        frame #0 {
          n345 = global read "QC_MeasurementSetup.vi" "CV Measurement Parameters"() -> (w549:T7)
          n346 = Unbundle By Name(w549) -> ("V_depletion Limit [V]"=w541:dbl, "Number Of Steps"=w544:u32)
          n347 = case shown="True" w539 {
            tunnel: ["" w575] -> w550
            tunnel: [_ w558] -> w548
            tunnel: w544 -> [_ w555]
            frame False {
            }
            frame True {
              w556 = T3."Read Array" ("Action")
              n348 = local write "STATUS 1"("Saving Data ...") -> ()
              n349 = call "CVData.vi"("Action"=w556, "Array No."=u32 4 ("Action")) -> ("Array OUT"=w571:dbl[])  [unwired: 3 in, 1 out]
              n350 = call "CVData.vi"("Action"=w556, "Array No."=u32 3 ("Action")) -> ("Array OUT"=w570:dbl[])  [unwired: 3 in, 1 out]
              n351 = call "CVData.vi"("Action"=w556, "Array No."=u32 2 ("Action")) -> ("Array OUT"=w553:dbl[])  [unwired: 3 in, 1 out]
              n352 = call <vilib>:"Std Deviation and Variance.vi"("X"=w571) -> ("mean"=w559:dbl)  [unwired: 1 in, 2 out]
              n353 = call <vilib>:"Std Deviation and Variance.vi"("X"=w570) -> ("mean"=w560:dbl)  [unwired: 1 in, 2 out]
              n354 = Multiply(x=w553, y=0.001) -> (x*y=w552:dbl[])
              n355 = call "CVData.vi"("Action"=w556, "Array No."=u32 0 ("Action")) -> ("Array OUT"=w565:dbl[])  [unwired: 3 in, 1 out]
              n356 = call "CVData.vi"("Action"=w556, "Array No."=u32 1 ("Action")) -> ("Array OUT"=w564:dbl[])  [unwired: 3 in, 1 out]
              n357 = Build Array(w565, w564, w552) -> (w563:dbl[][])
              n358 = Transpose 2D Array(2D array=w563) -> (transposed array=w562:dbl[][])
              n359 = call "SaveDataFile.vi"("Arrays format"="%010.2f", "Humidity"=w559, "Array Titles"="Voltage[V] Capacitance[pF] Resistance[kOhm]", "Temperature"=w560, "Actual array lengths"=w555, "no. of arrays"=3, "Data Array"=w562) -> ("Error Out"=w558:errorcluster, "Path + Filename OUT"=w575:string)  [unwired: 1 in, 2 out]
            }
          }
          n360 = Absolute Value(x=w541) -> (abs(x)=w540:dbl)
          n361 = call "ScanFeedback.vi"("measurement type"=T2."CV") -> ("V depletion"=w543:dbl)  [unwired: 3 in, 5 out]
          n362 = Absolute Value(x=w543) -> (abs(x)=w542:dbl)
          n363 = Less Or Equal?(x=w542, y=w540) -> (x <= y?=w545:bool)
          n364 = call "WriteLogFile.vi"("Data File"=w550, "Error In"=w548, "DUT passed?"=w545, "Value TechSpec criteria"=w543, "Files saved?"=w539) -> ()  [unwired: 6 in, 1 out]
        }
      }
      n365 = Select(t="Run finished.\nData saved." ("STATUS 1"), s=w527, f="Run finished.\nData not saved." ("STATUS 1")) -> (s? t:f=w530:string)
      n366 = local write "STATUS 1"(w530) -> ()
      "Done!" <- w525
    }
  }
